vi "Complex SVD Factorization.vi"(0 "A":T1) -> (1 "U":T1, 2 "S":cdb[](array[numeric]), 3 "V":T1, 4 "error":i32)   [LabVIEW 2017, in "NI_AALPro.lvlib"]
doc: "Performs the singular value decomposition (SVD) of a given m-by-n, complex matrix <B>A</B>. The dimentions of U, S, and V are m x min(m, n), min(m, n), and n x min(m, n), respectively."
uses:
  NI_AALPro.lvlib
  ComplexMatrix.ctl
  lvanlys.dll
  NI_Matrix.lvlib
panel:
  # "Complex SVD Factorization"
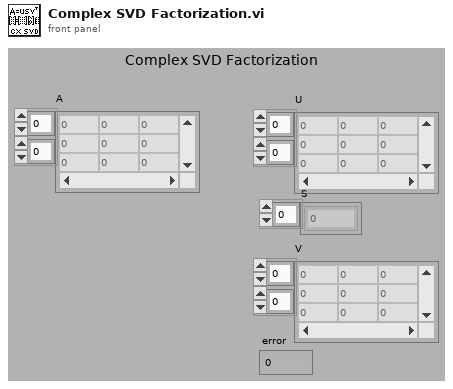
[diagram p1: front panel]
types:
  T1 = typedef "NI_Matrix.lvlib/ComplexMatrix.ctl" = cdb[][]
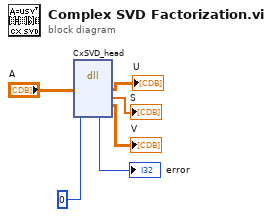
[diagram p0: block diagram]
diagram:
  n1 = dll-call lib="C:/Program Files/National Instruments/LabVIEW 2017/resource/lvanlys.*" fn="CxSVD_head"("A"="A", 0) -> ("A"=→"U":T1, "S"=→"S":cdb[], "V"=→"V":T1, →"error":i32)  [unwired: 6 in, 2 out]
